vi "GraphWrite.vi"(7 "LabVIEW Web Service Request":refnum<class "Web Request.lvclass">) -> ()   [LabVIEW 2018]
uses:
  <vilib>/wsapi/Web Request.lvclass
  Lib/STM/Graph/MOKO_Graph_main_ITEM.ctl
  Lib/STM/Graph/MOKO_Graph_main_STM.ctl
panel:
  out "error out":errorcluster
  # "Use the Web Service Request input terminal to call the VIs on the Web Services palette. Do not remove it from the connector pane unless you don't need access to the palette."
  # "Each additional control wired to the connector pane will be available as an input in the URL. To include an indicator in terminal-mode output (the default setting), it must also be wired to the connector pane."
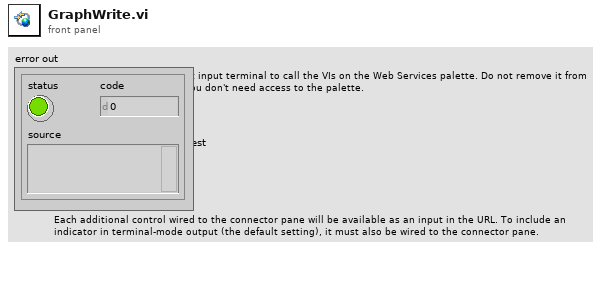
[diagram p1: front panel]
types:
  T1 = typedef "MOKO_Graph_main_ITEM.ctl" = enum16{"idle", "Graph read", "Graph write"}
  T2 = typedef "MOKO_Graph_main_STM.ctl" = cluster{"main stm":T1, "data":string}
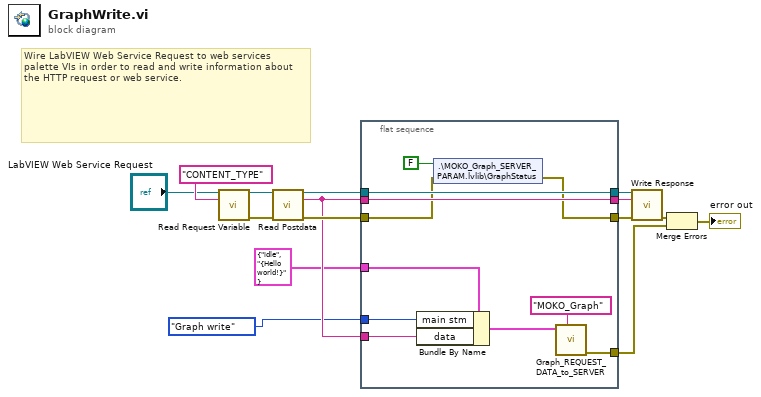
[diagram p0: block diagram]
diagram:
  # "Wire LabVIEW Web Service Request to web services palette VIs in order to read and write information about the HTTP request or web service."
  n1 = call <vilib>:"Read Request Variable.vi"("LabVIEW Web Service Request"="LabVIEW Web Service Request", "variable name"="CONTENT_TYPE") -> ("LabVIEW Web Service Request out"=w14:refnum<class "Web Request.lvclass">, "error out"=w13:errorcluster)  [unwired: 11 in, 1 out]
  n2 = call <vilib>:"Read Postdata.vi"("LabVIEW Web Service Request"=w14, "error in (no error)"=w13) -> ("LabVIEW Web Service Request out"=w6:refnum<class "Web Request.lvclass">, "postdata"=w8:string, "error out"=w9:errorcluster)  [unwired: 11 in]
  n3 = flat-sequence {
    tunnel: w8 -> [w26]
    tunnel: T2 {"main stm"=enum."idle", "data"="{Hello world!}"} ("MOKO_NMEA_STM") -> [w24]
    tunnel: [w23] -> w10
    tunnel: w9 -> [w18]
    tunnel: w8 -> [w22]
    tunnel: [w22] -> w7
    tunnel: w6 -> [w21]
    tunnel: [w21] -> w5
    tunnel: [w17] -> w4
    tunnel: MOKO_Graph_main_ITEM."Graph write" ("main stm") -> [w16]
    frame #0 {
      n4 = Bundle By Name(cluster=w24, "main stm"=w16, "data"=w26) -> (w20:T2)
      n5 = shared-variable ".\\MOKO_Graph_SERVER_PARAM.lvlib\\GraphStatus"(FALSE, error in=w18) -> (error out=w17:errorcluster)
      n6 = call "Graph_REQUEST_DATA_to_SERVER.vi"("Control Name"="MOKO_Graph", "MOKO_ExPlugin_STM"=w20) -> ("Error Out"=w23:errorcluster)  [unwired: 9 in]
    }
  }
  n7 = call <vilib>:"Write Response.vi"("LabVIEW Web Service Request"=w5, "response string"=w7, "error in (no error)"=w4) -> ("error out"=w12:errorcluster)  [unwired: 11 in, 1 out]
  n8 = Merge Errors(w12, w10) -> (→"error out":errorcluster)
